vi "Hahn 1 Pulse Sequence Generator.vi"(0 "Pulse offset":dbl, 4 "Equal Pulse length":bool, 5 "Array":T1(array[cluster]), 6 "MW Delay":dbl, 7 "No. Instructions":i32, 8 "Tau step size":dbl, 9 "Tau max":dbl, 10 "Tau min":dbl, 11 "Rabi Frequency":dbl) -> (2 "Tau":dbl[](array[numeric]), 3 "Pulse Sequence":T1(array[cluster]))   [LabVIEW 2012]
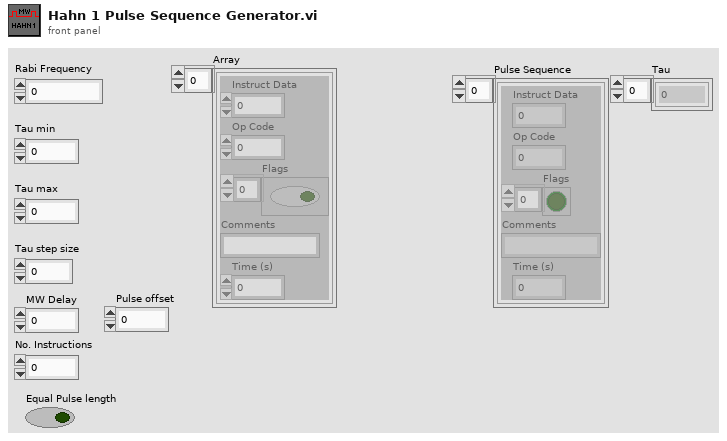
[diagram p1: front panel]
types:
  T1 = cluster{"Instruct Data":i32, "Op Code":i32, "Flags":bool[], "Comments":string, "Time (s)":dbl}[]
  T2 = cluster{"Instruct Data":i32, "Op Code":i32, "Flags":bool[], "Comments":string, "Time (s)":dbl}
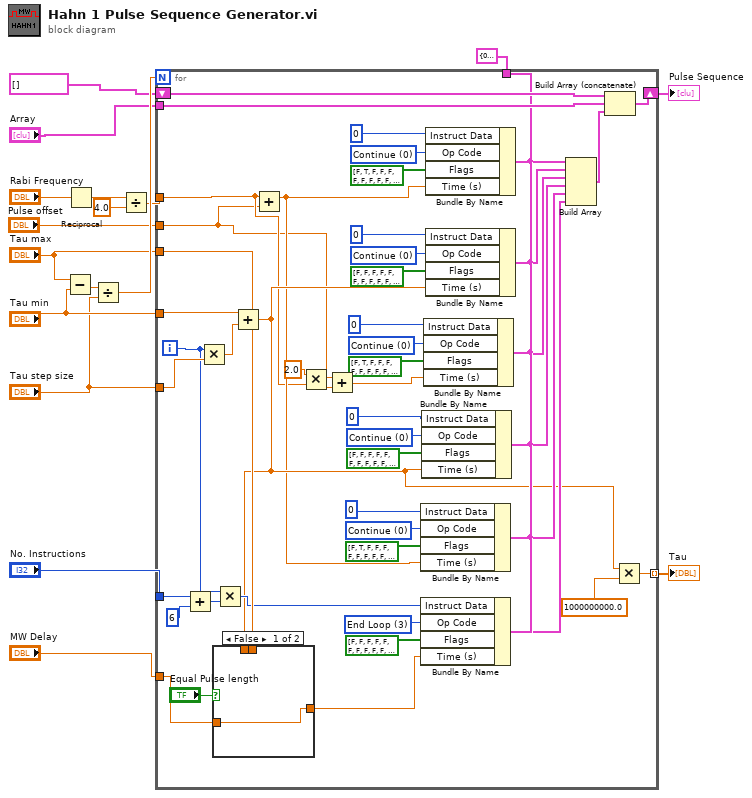
[diagram p0: block diagram]
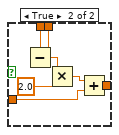
[diagram p2: hidden frame]
diagram:
  n1 = Subtract(x="Tau max", y="Tau min") -> (x-y=w17:dbl)
  n2 = Reciprocal(x="Rabi Frequency") -> (1/x=w14:dbl)
  n3 = Divide(x=w17, y="Tau step size") -> (x/y=w16:dbl)
  n4 = Divide(x=w14, y=4.0) -> (x/y=w13:dbl)
  n5 = for {
    N: w16 -> [_]
    tunnel: w13 -> [w20]
    tunnel: "Tau max" -> [w40]
    tunnel: "Tau min" -> [w57]
    tunnel: "Tau step size" -> [w56]
    shift-right: [w63] -> w3
    shift-left: T1 [] -> [w62]
    tunnel: "Array" -> [w61]
    tunnel: T2 {"Instruct Data"=0, "Op Code"=0, "Flags"=[FALSE, FALSE, FALSE, FALSE, FALSE, FALSE, FALSE, FALSE, FALSE, FALSE, FALSE, FALSE, FALSE, FALSE, FALSE, FALSE, FALSE, FALSE, FALSE, FALSE, FALSE, TRUE, TRUE, TRUE], "Comments"="", "Time (s)"=0.01} ("PB Inst 2") -> [w41]
    tunnel: "MW Delay" -> [w24]
    tunnel: "No. Instructions" -> [w38]
    tunnel: [w25] -> w2 mode=indexing
    tunnel: "Pulse offset" -> [w18]
    i -> [w36]
    w42 = 3 items=["Continue", "Stop", "Loop", "End Loop", "JSR", "RTS", "Branch", "Long Delay", "Wait"] ("Op Code")
    w45 = 0 items=["Continue", "Stop", "Loop", "End Loop", "JSR", "RTS", "Branch", "Long Delay", "Wait"] ("Op Code")
    w48 = 0 items=["Continue", "Stop", "Loop", "End Loop", "JSR", "RTS", "Branch", "Long Delay", "Wait"] ("Op Code")
    w53 = 0 items=["Continue", "Stop", "Loop", "End Loop", "JSR", "RTS", "Branch", "Long Delay", "Wait"] ("Op Code")
    w59 = 0 items=["Continue", "Stop", "Loop", "End Loop", "JSR", "RTS", "Branch", "Long Delay", "Wait"] ("Op Code")
    w65 = 0 items=["Continue", "Stop", "Loop", "End Loop", "JSR", "RTS", "Branch", "Long Delay", "Wait"] ("Op Code")
    n6 = Add(x=w38, y=6) -> (x+y=w37:i32)
    n7 = Multiply(x=w36, y=w56) -> (x*y=w55:dbl)
    n8 = Multiply(x=w36, y=w37) -> (x*y=w35:i32)
    n9 = Add(x=w57, y=w55) -> (x+y=w26:dbl)
    n10 = case shown="False" "Equal Pulse length" {
      tunnel: w40 -> [_ w74]
      tunnel: w26 -> [_ w71]
      tunnel: w24 -> [w67 w69]
      tunnel: [w67 w68] -> w23
      frame False {
      }
      frame True {
        n11 = Subtract(x=w74, y=w71) -> (x-y=w73:dbl)
        n12 = Multiply(x=w73, y=2.0) -> (x*y=w70:dbl)
        n13 = Add(x=w70, y=w69) -> (x+y=w68:dbl)
      }
    }
    n14 = Add(x=w20, y=w18) -> (x+y=w21:dbl)
    n15 = Multiply(x=2.0, y=w20) -> (x*y=w51:dbl)
    n16 = Add(x=w18, y=w51) -> (x+y=w19:dbl)
    n17 = Bundle By Name(cluster=w41, "Instruct Data"=0, "Op Code"=w45, "Flags"=bool[] [FALSE, TRUE, FALSE, FALSE, FALSE, FALSE, FALSE, FALSE, FALSE, FALSE, FALSE, FALSE, FALSE, FALSE, FALSE, FALSE, FALSE, FALSE, FALSE, FALSE, FALSE, TRUE, TRUE, TRUE], "Time (s)"=w21) -> (w31:T2)
    n18 = Bundle By Name(cluster=w41, "Instruct Data"=w35, "Op Code"=w42, "Flags"=bool[] [FALSE, FALSE, FALSE, FALSE, FALSE, FALSE, FALSE, FALSE, FALSE, FALSE, FALSE, FALSE, FALSE, FALSE, FALSE, FALSE, FALSE, FALSE, FALSE, FALSE, FALSE, TRUE, TRUE, TRUE], "Time (s)"=w23) -> (w32:T2)
    n19 = Bundle By Name(cluster=w41, "Instruct Data"=0, "Op Code"=w48, "Flags"=bool[] [FALSE, FALSE, FALSE, FALSE, FALSE, FALSE, FALSE, FALSE, FALSE, FALSE, FALSE, FALSE, FALSE, FALSE, FALSE, FALSE, FALSE, FALSE, FALSE, FALSE, FALSE, TRUE, TRUE, TRUE], "Time (s)"=w26) -> (w30:T2)
    n20 = Bundle By Name(cluster=w41, "Instruct Data"=0, "Op Code"=w53, "Flags"=bool[] [FALSE, TRUE, FALSE, FALSE, FALSE, FALSE, FALSE, FALSE, FALSE, FALSE, FALSE, FALSE, FALSE, FALSE, FALSE, FALSE, FALSE, FALSE, FALSE, FALSE, FALSE, TRUE, TRUE, TRUE], "Time (s)"=w19) -> (w29:T2)
    n21 = Bundle By Name(cluster=w41, "Instruct Data"=0, "Op Code"=w65, "Flags"=bool[] [FALSE, TRUE, FALSE, FALSE, FALSE, FALSE, FALSE, FALSE, FALSE, FALSE, FALSE, FALSE, FALSE, FALSE, FALSE, FALSE, FALSE, FALSE, FALSE, FALSE, FALSE, TRUE, TRUE, TRUE], "Time (s)"=w21) -> (w33:T2)
    n22 = Bundle By Name(cluster=w41, "Instruct Data"=0, "Op Code"=w59, "Flags"=bool[] [FALSE, FALSE, FALSE, FALSE, FALSE, FALSE, FALSE, FALSE, FALSE, FALSE, FALSE, FALSE, FALSE, FALSE, FALSE, FALSE, FALSE, FALSE, FALSE, FALSE, FALSE, TRUE, TRUE, TRUE], "Time (s)"=w26) -> (w28:T2)
    n23 = Build Array(w33, w28, w29, w30, w31, w32) -> (w34:T1)
    n24 = Build Array (concatenate)(w62, w61, w34) -> (w63:T1)
    n25 = Multiply(x=w26, y=1000000000.0) -> (x*y=w25:dbl)
  }
  "Pulse Sequence" <- w3
  "Tau" <- w2
